vi "Check Convention.vi"(1 "terminal name array":string[](array[string])) -> (0 "validation result":string="All terminal names are formal")   [LabVIEW 2016]
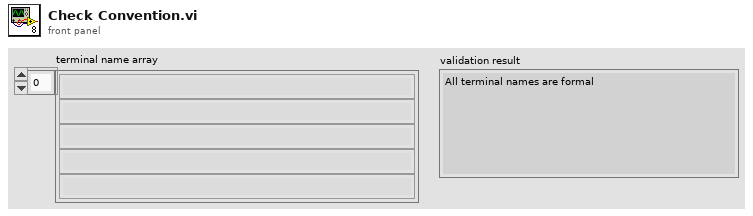
[diagram p1: front panel]
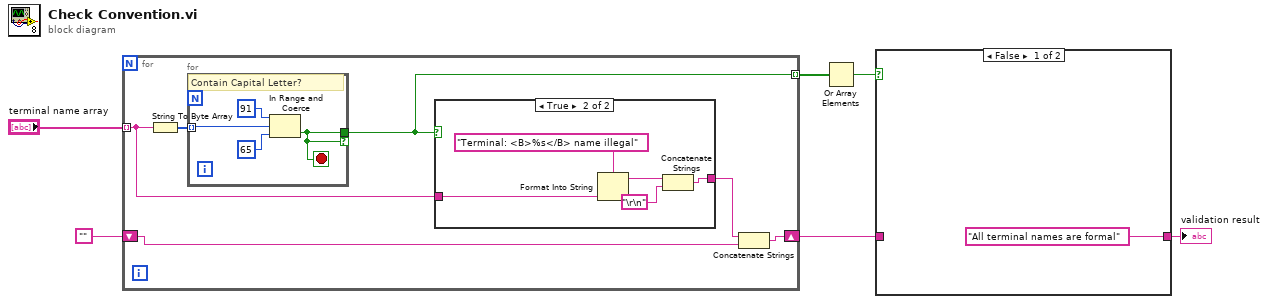
[diagram p0: block diagram]
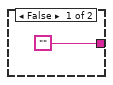
[diagram p3: hidden frame]
diagram:
  n1 = for {
    tunnel: "terminal name array" -> [w11] mode=indexing
    shift-right: [w10] -> w3
    shift-left: "" -> [w7]
    tunnel: [w9] -> w1 mode=indexing
    n2 = String To Byte Array(string=w11) -> (unsigned byte array=w12:u8[])
    n3 = for {
      tunnel: w12 -> [w22] mode=indexing
      tunnel: [w19] -> w9 if=w19
      stop <- w19 stop-if-true
      # "Contain Capital Letter?"
      n4 = In Range and Coerce(upper limit=u8 91, x=w22, lower limit=u8 65) -> (In Range?=w19:bool)  [unwired: 1 out]
    }
    n5 = case shown="True" w9 {
      tunnel: w11 -> [_ w16]
      tunnel: ["" w15] -> w8
      frame False {
      }
      frame True {
        n6 = Format Into String(format string="Terminal: <B>%s</B> name illegal", w16) -> (resulting string=w18:string)  [unwired: 2 in, 1 out]
        n7 = Concatenate Strings(w18, "\r\n") -> (w15:string)
      }
    }
    n8 = Concatenate Strings(w8, w7) -> (w10:string)
  }
  n9 = Or Array Elements(Boolean array=w1) -> (logical OR=w4:bool)
  n10 = case shown="False" w4 {
    tunnel: ["All terminal names are formal" w24] -> w2
    tunnel: w3 -> [_ w24]
    frame False {
    }
    frame True {
    }
  }
  "validation result" <- w2
